vi "FileExplorer.vi"() -> ()   [LabVIEW 2017]
uses:
  <vilib>/FTP/NI_FTP.lvlib
panel:
  out "error kopieren":errorcluster caption="Fehler (Ausgang)"
  in  "local path":path caption="Lokaler Pfad"
  in  "kopieren":bool
  in  "löschen":bool
  out "Numeric":i32
  out "error löschen":errorcluster
  out "filenames":string[](array[string])
  out "folder names":string[](array[string])
  out "error out":errorcluster
  in  "path":path
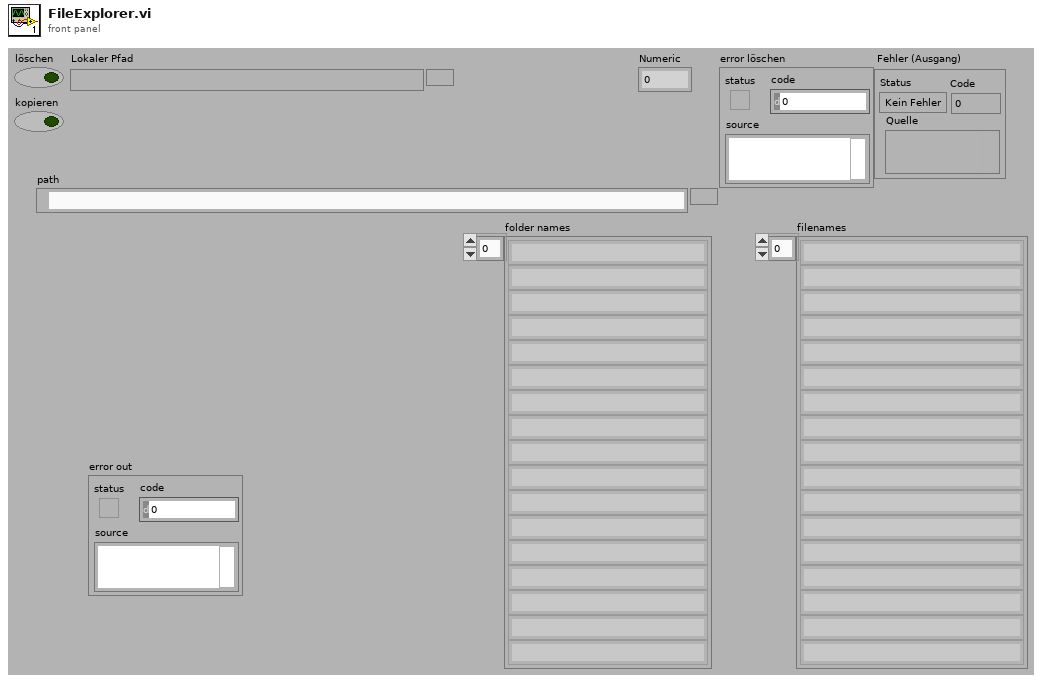
[diagram p1: front panel]
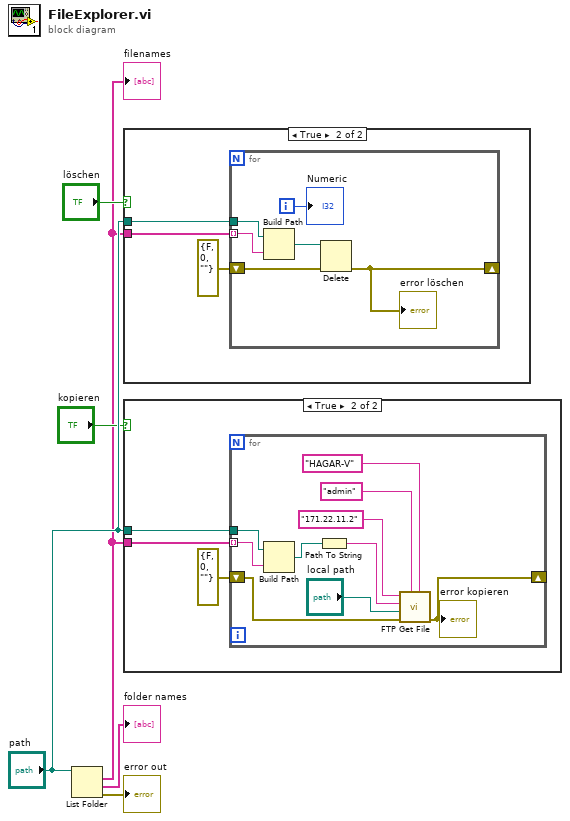
[diagram p0: block diagram]
diagram:
  n1 = List Folder(path="path") -> (filenames=w1:string[], folder names=→"folder names":string[], error out=→"error out":errorcluster)  [unwired: 3 in, 1 out]
  "filenames" <- w1
  n2 = case shown="True" "löschen" {
    tunnel: w1 -> [_ w9]
    tunnel: "path" -> [_ w8]
    frame False {
    }
    frame True {
      n3 = for {
        tunnel: w9 -> [w14] mode=indexing
        tunnel: w8 -> [w15]
        shift-right: [w12] -> _
        shift-left: errorcluster {"status"=FALSE, "code"=0, "source"=""} ("error out") -> [w11]
        i -> [w10]
        n4 = Build Path(base path=w15, name or relative path=w14) -> (appended path=w13:path)
        n5 = Delete(path (use dialog)=w13, error in=w11) -> (error out=w12:errorcluster)  [unwired: 3 in, 2 out]
        "error löschen" <- w12
        "Numeric" <- w10
      }
    }
  }
  n6 = case shown="True" "kopieren" {
    tunnel: "path" -> [_ w18]
    tunnel: w1 -> [_ w17]
    frame False {
    }
    frame True {
      n7 = for {
        shift-right: [w23] -> _
        shift-left: errorcluster {"status"=FALSE, "code"=0, "source"=""} ("error out") -> [w22]
        tunnel: w18 -> [w28]
        tunnel: w17 -> [w27] mode=indexing
        n8 = Build Path(base path=w28, name or relative path=w27) -> (appended path=w26:path)
        n9 = Path To String(path=w26) -> (string=w25:string)
        n10 = call <vilib>:"FTP Get File.vi"("password"="HAGAR-V", "user"="admin", "error in (no error)"=w22, "local path"="local path", "remote path"=w25, "host"="171.22.11.2") -> ("error out"=w23:errorcluster)  [unwired: 4 in, 1 out]
        "error kopieren" <- w23
      }
    }
  }
